vi "RH_PPMU_Close.vi"(8 "error in":errorcluster, 10 "Reset":bool, 11 "PPMU Session In":refnum<k15>) -> (0 "error out":errorcluster)   [LabVIEW 2023, in "ResourceHandling.lvlib"]
doc: "Disconnects all chassnels and close the session. Eventually it can Reset the device as well"
uses:
  ResourceHandling.lvlib
  <instrlib>/niDigital/niDigital.llb/niDigital Selected Function.ctl
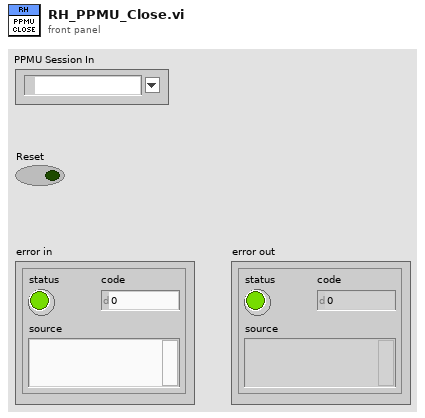
[diagram p1: front panel]
types:
  T1 = typedef "niDigital Selected Function.ctl" = i32
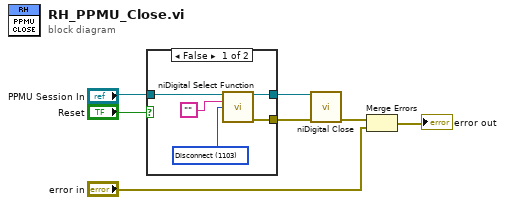
[diagram p0: block diagram]
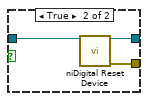
[diagram p2: hidden frame]
diagram:
  n1 = case shown="False" "Reset" {
    tunnel: "PPMU Session In" -> [w10 w15]
    tunnel: [w12 w14] -> w5
    tunnel: [w8 w13] -> w4
    frame False {
      w11 = T1 1103 items=["Digital"=1100, "PPMU"=1101, "Off"=1102, "Disconnect"=1103] ("function")
      n2 = call <instrlib>:"niDigital Select Function.vi"("instrument handle"=w10, "channel list"="", "function"=w11) -> ("instrument handle out"=w12:refnum<k15>, "error out"=w8:errorcluster)  [unwired: 11 in]
    }
    frame True {
      n3 = call <instrlib>:"niDigital Reset Device.vi"("instrument handle in"=w15) -> ("instrument handle out"=w14:refnum<k15>, "error out"=w13:errorcluster)  [unwired: 13 in]
    }
  }
  n4 = call <instrlib>:"niDigital Close.vi"("instrument handle"=w5, "error in"=w4) -> ("error out"=w7:errorcluster)  [unwired: 13 in]
  n5 = Merge Errors(w7, "error in") -> (→"error out":errorcluster)
